vi "AutoTemp.vi"(0 "Database":T2={"DB name"="zaop", "UID"="jdennis", "password"=""}, 1 "Z Address":T1, 2 "Log file":path=path "nologfile", 5 "measSetId list":string="1", 9 "Comment(SN)":string, 12 "CW":bool) -> (6 "measResId table":i32[](array[numeric]), 15 "error out":errorcluster)   [LabVIEW 2016]
doc: "This program executes a list of intensity measurements for different Z system settings. Given a list of measSetId for the measurements to be made, the program first retrieves the corresponding measurement conditions from the database, along with accessory parameters (specified by measIntenParamId, measSSId). An interrupt window is displayed for a user to reorder/stop measurements, and measurements are run using MeasOneSetZ.vi. After each one, PickNextMeasZ.vi is used to select the next measurement. After the measurements end, the result IDs (measResId) and any errors or warnings are displayed, and the user can alter the value of \"isDataUsable\" in the database."
uses:
  type def/ZAddress.ctl
  type def/Database.ctl
  user/GrobaLimitVoltage.vi
panel:
  in  "read reps":i16=5
  in  "spotcheck interval":u16=20
  in  "allowed reps":u16=1
  in  "error in (no error)":errorcluster
  # "Inputs"
  # "Outputs"
  # "Program constants"
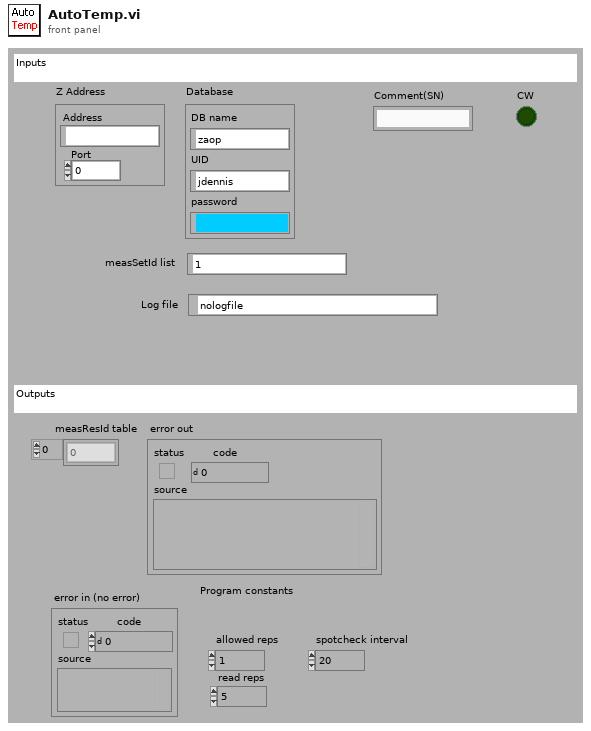
[diagram p1: front panel]
types:
  T1 = typedef "ZAddress.ctl" = cluster{"Address":string, "Port":u16}
  T2 = typedef "Database.ctl" = cluster{"DB name":string, "UID":string, "password":string}
  T3 = cluster{"curr index":u16, "next index":u16, "num reps":u16, "allowed rep":u16, "SC count":u16, "SC interval":u16}
  T4 = typedef "measSetting.ctl" = cluster{"measSetId":i32, "measSetComments":string, "probeId":sgl, "beamstyleIndex":i16, "txFrequencyHz":sgl, "focusRangeCm":sgl, "maxTxVoltageVolt":sgl, "ceilTxVoltageVolt":sgl, "profTxVoltageVolt":dbl, "totalVoltagePt":i8, "numMeasVoltage":i8, "numTxElements":i16, "txpgWaveformStyle":i8, "numTxCycles":sgl, "elevAperIndex":i8, "zStartDistCm":sgl, "zMeasNum":i8, "IsTxAperModulationEn":i8, "DTxFreqIndex":i16, "VTxIndex":i8, "IsCPAEn":i16, "SysPulserSelA":i16, "TxPulseRleA":string}
  T5 = cluster{"measSetId":i32, "measResId":i32, "errors":string[], "status":bool}[]
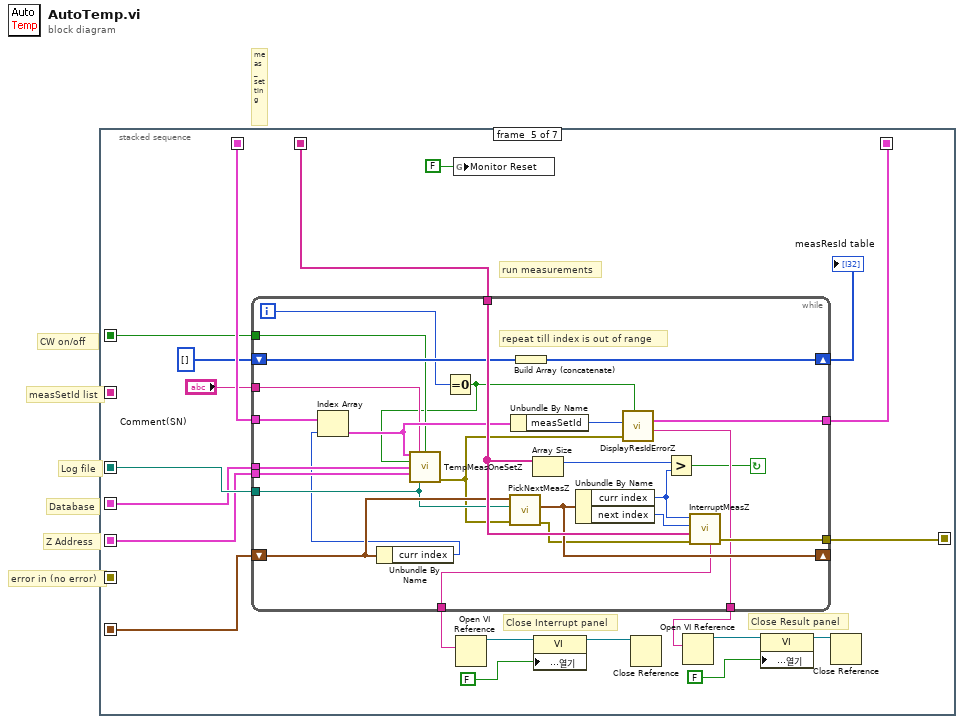
[diagram p0: block diagram]
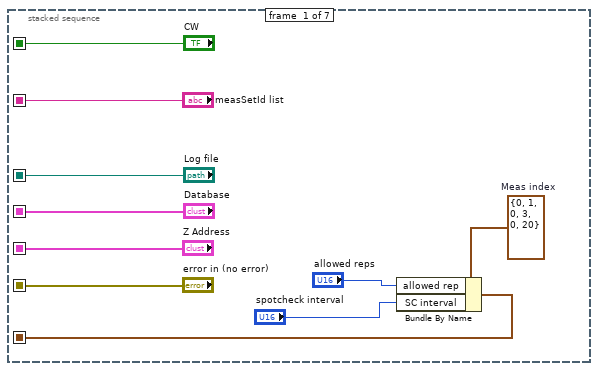
[diagram p2: hidden frame]
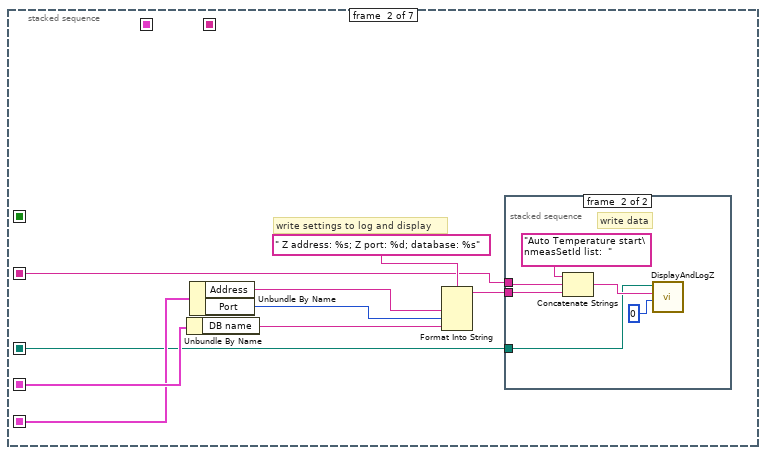
[diagram p3: hidden frame]
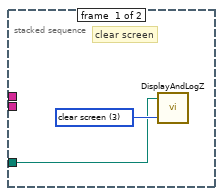
[diagram p4: hidden frame]
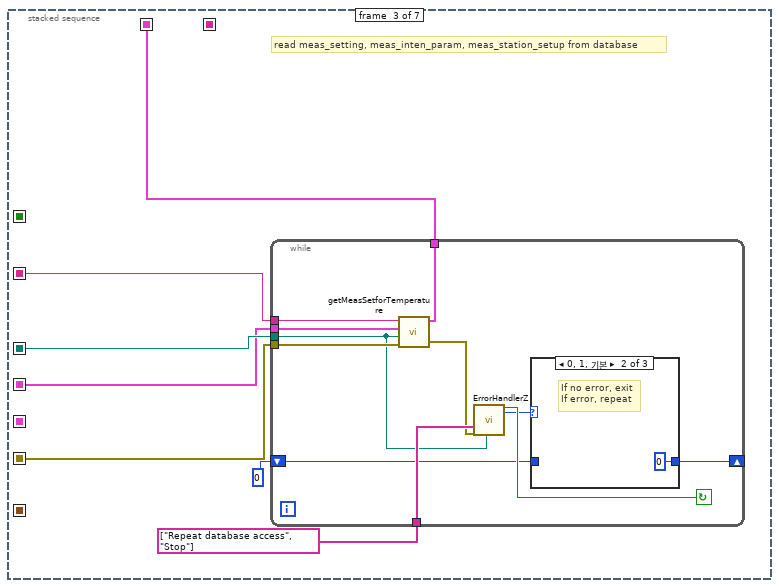
[diagram p5: hidden frame]
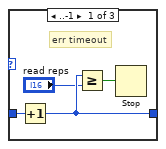
[diagram p6: hidden frame]
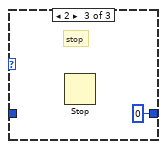
[diagram p7: hidden frame]
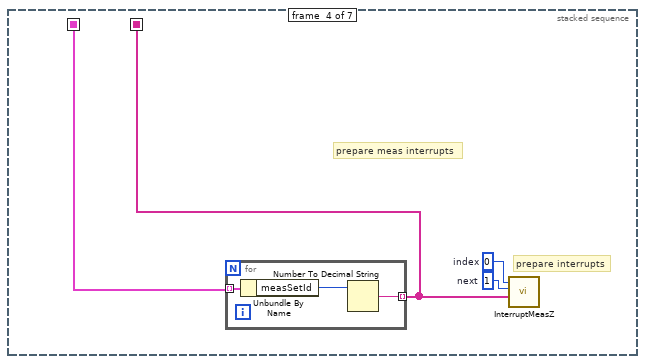
[diagram p8: hidden frame]
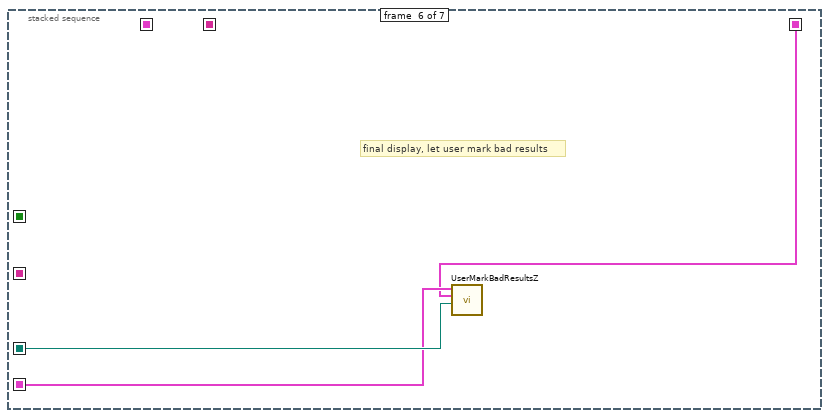
[diagram p9: hidden frame]
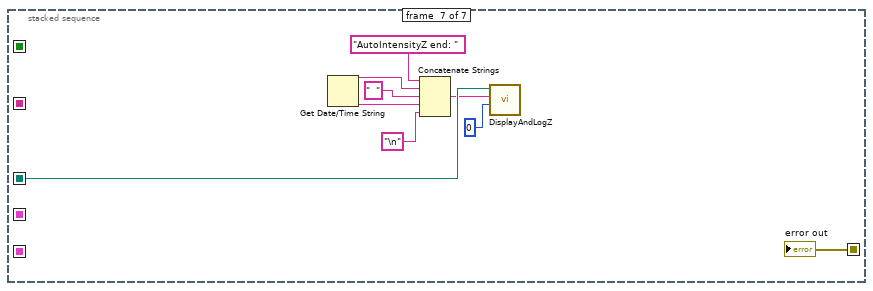
[diagram p10: hidden frame]
diagram:
  # "meas_setting"
  # "error in (no error)"
  # "Z Address"
  # "Database"
  # "Log file"
  # "measSetId list"
  # "CW on/off"
  n1 = stacked-sequence {
    seq-local: [_ _ w34 _ _ _ _] -> [_ _ _ w54 w79 _ _]
    seq-local: [_ _ _ w55 _ _ _] -> [_ _ _ _ w78 _ _]
    seq-local: ["measSetId list" _ _ _ _ _ _] -> [_ w17 w33 _ _ _ _]
    seq-local: ["Log file" _ _ _ _ _ _] -> [_ w14 w32 _ w77 w108 w117]
    seq-local: ["Database" _ _ _ _ _ _] -> [_ w16 w31 _ w76 w107 _]
    seq-local: ["Z Address" _ _ _ _ _ _] -> [_ w15 _ _ w75 _ _]
    seq-local: ["error in (no error)" _ _ _ _ _ _] -> [_ _ w30 _ _ _ _]
    seq-local: [w2 _ _ _ _ _ _] -> [_ _ _ _ w72 _ _]
    seq-local: [_ _ _ _ w74 _ _] -> [_ _ _ _ _ w106 _]
    seq-local: [_ _ _ _ w73 _ _] -> [_ _ _ _ _ _ w116]
    seq-local: ["CW" _ _ _ _ _ _] -> [_ _ _ _ w59 _ _]
    frame #0 {
      w5 = T3 {"curr index"=0, "next index"=1, "num reps"=0, "allowed rep"=3, "SC count"=0, "SC interval"=20}  # Meas index
      n2 = Bundle By Name(cluster=w5, "allowed rep"="allowed reps", "SC interval"="spotcheck interval") -> (w2:T3)
    }
    frame #1 {
      # "write settings to log and display"
      n3 = Unbundle By Name(w16) -> ("DB name"=w11:string)
      n4 = Unbundle By Name(w15) -> ("Address"=w13:string, "Port"=w12:u16)
      n5 = Format Into String(format string=" Z address: %s; Z port: %d; database: %s" ("Format String"), w13, w12, w11) -> (resulting string=w18:string)  [unwired: 2 in, 1 out]
      n6 = stacked-sequence {
        tunnel: w18 -> [_ w24]
        tunnel: w17 -> [_ w23]
        tunnel: w14 -> [w20 w22]
        frame #0 {
          w21 = u16 3 items=["to file + screen", "to file", "to screen", "clear screen"] ("action")
          # "clear screen"
          n7 = call "DisplayAndLogZ.vi"("Log file"=w20, "action (0: log+display)"=w21) -> ()  [unwired: 6 in, 1 out]
        }
        frame #1 {
          # "write data"
          n8 = Concatenate Strings("Auto Temperature start\nmeasSetId list:  " ("Substring"), w23, w24) -> (w25:string)
          n9 = call "DisplayAndLogZ.vi"("Log file"=w22, "message"=w25, "action (0: log+display)"=u16 0) -> ()  [unwired: 5 in, 1 out]
        }
      }
    }
    frame #2 {
      # "read meas_setting, meas_inten_param, meas_station_setup from database"
      n10 = while {
        shift-left: i16 0 -> [w42]
        shift-right: [w41] -> _
        tunnel: [w39] -> w34
        tunnel: w31 -> [w37]
        tunnel: string[] ["Repeat database access", "Stop"] ("dialog prompts") -> [w44]
        tunnel: w30 -> [w45]
        tunnel: w32 -> [w38]
        tunnel: w33 -> [w40]
        stop <- w43 continue-if-true
        n11 = call "getMeasSetforTemperature.vi"("measSetId"=w40, "Database"=w37, "Log file"=w38, "error in (no error)"=w45) -> ("meas_setting array"=w39:T4[], "error out"=w35:errorcluster)  [unwired: 5 in]
        n12 = call "ErrorHandlerZ.vi"("dialog prompts"=w44, "error in (no error)"=w35, "Log file"=w38) -> ("selection/timeout (0)"=w36:i16, "error?"=w43:bool)  [unwired: 11 in, 4 out]
        n13 = case shown="0, 1, 기본" w36 {
          tunnel: w42 -> [w49 _ _]
          tunnel: [w48 i16 0 i16 0] -> w41
          frame ..-1 {
            # "err timeout"
            n14 = Increment(x=w49) -> (x+1=w48:i16)
            n15 = Greater Or Equal?(x=w48, y="read reps") -> (x >= y?=w47:bool)
            n16 = Stop(stop? (T)=w47) -> ()
          }
          frame 0, 1, Default {
            # "If no error, exit\nIf error, repeat"
          }
          frame 2 {
            # "stop"
            n17 = Stop() -> ()  [unwired: 1 in]
          }
        }
      }
    }
    frame #3 {
      w52 = u16 1  # next
      w53 = u16 0  # index
      # "prepare meas interrupts"
      # "prepare interrupts"
      n18 = for {
        tunnel: w54 -> [w58] mode=indexing
        tunnel: [w56] -> w55 mode=indexing
        n19 = Unbundle By Name(w58) -> ("measSetId"=w57:i32)
        n20 = Number To Decimal String(number=w57) -> (decimal integer string=w56:string)  [unwired: 1 in]
      }
      n21 = call "InterruptMeasZ.vi"("meas_id"=w55, "next index"=w52, "current index"=w53) -> ()  [unwired: 4 in, 5 out]
    }
    frame #4 {
      # "Close Result panel"
      # "Close Interrupt panel"
      # "run measurements"
      n22 = while {
        tunnel: [w95] -> w63
        tunnel: [w96] -> w74
        tunnel: [w100] -> w71
        shift-left: w72 -> [w94]
        shift-right: [w101] -> _
        tunnel: [w102] -> w73
        tunnel: w76 -> [w99]
        tunnel: w75 -> [w98]
        shift-left: i32[] [] ("measResId table def") -> [w103]
        shift-right: [w97] -> w67
        tunnel: w79 -> [w105]
        tunnel: w78 -> [w104]
        tunnel: w77 -> [w93]
        tunnel: "Comment(SN)" -> [w82]
        tunnel: w59 -> [w81]
        i -> [w92]
        stop <- w91 continue-if-true
        # "repeat till index is out of range"
        n23 = Unbundle By Name(w94) -> ("curr index"=w89:u16)
        n24 = Index Array(array=w105, index=w89) -> (element=w86:T4)
        n25 = Equal To 0?(x=w92) -> (x = 0?=w80:bool)
        n26 = call "TempMeasOneSetZ.vi"("meas_setting"=w86, "Comment(SN)"=w82, "CW"=w81, "initial \ncommand"=w80, "Database"=w99, "Z Address"=w98, "Log file"=w93) -> ("error out"=w84:errorcluster)  [unwired: 8 in]
        n27 = call "PickNextMeasZ.vi"("error in (no error)"=w84, "Log file"=w93, "Meas index"=w94) -> ("error out"=w90:errorcluster, "new Meas index"=w101:T3)  [unwired: 7 in]
        n28 = Unbundle By Name(w86) -> ("measSetId"=w85:i32)
        n29 = Build Array (concatenate)(w103) -> (w97:i32[])
        n30 = Array Size(array=w104) -> (size(s)=w83:i32)
        n31 = Unbundle By Name(w101) -> ("curr index"=w88:u16, "next index"=w87:u16)
        n32 = call "DisplayResIdErrorZ.vi"("First iteration"=w80, "error in (no error)"=w84, "measSetId"=w85) -> ("VI's path"=w95:string, "ID summary"=w96:T5)  [unwired: 4 in, 1 out]
        n33 = Greater?(x=w83, y=w88) -> (0:w91:bool)
        n34 = call "InterruptMeasZ.vi"("error in (no error)"=w90, "meas_id"=w104, "next index"=w87, "current index"=w88) -> ("error out"=w102:errorcluster, "VI's path"=w100:string)  [unwired: 3 in, 3 out]
      }
      "measResId table" <- w67
      n35 = global write "GrobaLimitVoltage.vi" "Monitor Reset"(FALSE ("Monitor Reset")) -> ()
      n36 = Open VI Reference(vi path=w71) -> (vi reference=w70:refnum<vi>)  [unwired: 5 in, 1 out]
      n37 = property class="VI"(reference=w70, "프런트패널 윈도우:열기"=FALSE ("Front Panel Window:Open")) -> (reference out=w68:refnum<vi>)  [unwired: 1 in, 1 out]
      n38 = Close Reference(reference=w68) -> ()  [unwired: 1 in, 1 out]
      n39 = Open VI Reference(vi path=w63) -> (vi reference=w66:refnum<vi>)  [unwired: 5 in, 1 out]
      n40 = property class="VI"(reference=w66, "프런트패널 윈도우:열기"=FALSE ("Front Panel Window:Open")) -> (reference out=w64:refnum<vi>)  [unwired: 1 in, 1 out]
      n41 = Close Reference(reference=w64) -> ()  [unwired: 1 in, 1 out]
    }
    frame #5 {
      # "final display, let user mark bad results"
      n42 = call "UserMarkBadResultsZ.vi"("Log file"=w108, "ID summary"=w106, "Database"=w107) -> ()  [unwired: 4 in, 1 out]
    }
    frame #6 {
      n43 = Get Date/Time String() -> (date string=w114:string, time string=w112:string)  [unwired: 3 in]
      n44 = Concatenate Strings("AutoIntensityZ end: " ("Substring"), w114, "  ", w112, "\n" ("Substring")) -> (w110:string)
      n45 = call "DisplayAndLogZ.vi"("Log file"=w117, "message"=w110, "action (0: log+display)"=u16 0) -> ()  [unwired: 5 in, 1 out]
      "error out" <- w116
    }
  }
